vi "FF_ReadTxtFile.vi"(8 "error in (no error)":errorcluster, 10 "Path":path, 11 "ForceField in":refnum<class "ForceField.lvclass">) -> (0 "error out":errorcluster, 2 "Array":dbl[][](array[numeric]), 3 "ForceField out":refnum<class "ForceField.lvclass">)   [LabVIEW 2015, in "ForceField.lvclass"]
uses:
  ForceField.lvclass
  <vilib>/Utility/file.llb/Read From Spreadsheet File (DBL).vi
panel:
  out "Waveform Graph":dbl[][](graph)
  in  "delimiter (\\t)":string=","
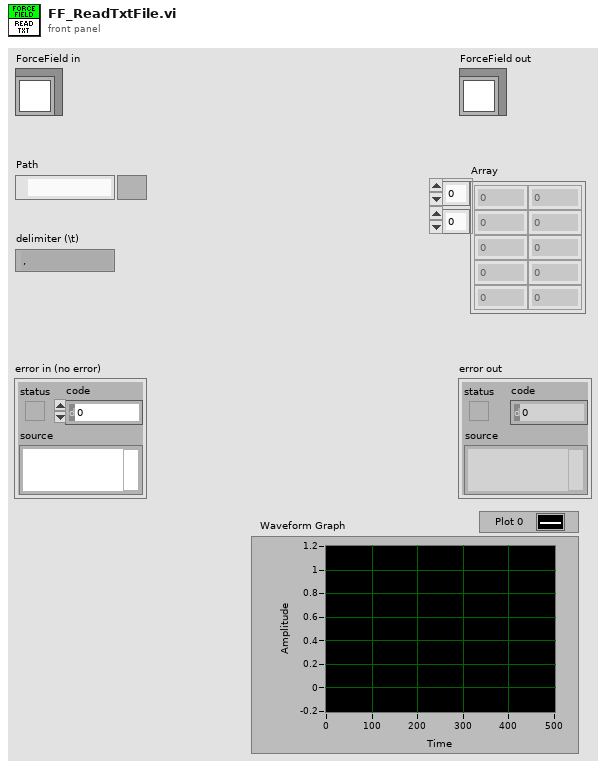
[diagram p1: front panel]
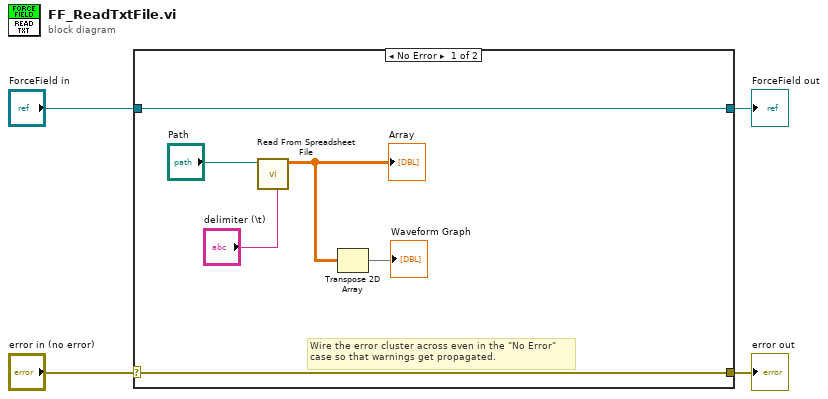
[diagram p0: block diagram]
diagram:
  n1 = case shown="No Error" "error in (no error)" {
    selector: "error in (no error)" -> [w9 w12]
    tunnel: [w9 w12] -> w3
    tunnel: [w10 w11] -> w1
    tunnel: "ForceField in" -> [w10 w11]
    frame No Error {
      # "Wire the error cluster across even in the \"No Error\"\ncase so that warnings get propagated."
      n2 = call-poly <vilib>:"Read From Spreadsheet File.vi"("delimiter (\\t)"="delimiter (\\t)", "file path (dialog if empty)"="Path") -> ("all rows"=w6:dbl[][])  [unwired: 5 in, 4 out]
      "Array" <- w6
      n3 = Transpose 2D Array(2D array=w6) -> (transposed array=→"Waveform Graph":dbl[][])
    }
    frame Error {
    }
  }
  "error out" <- w3
  "ForceField out" <- w1
